vi "Play with rts cts 1002759.vi"(8 "error in (no error)":errorcluster, 11 "Serial open? (y)":bool=TRUE) -> (0 "error out":errorcluster, 1 "RTS control ok?":bool, 3 "PassFail":string, 4 "Comport responsive?":bool, 5 "Comport unresponsive?":bool)   [LabVIEW 2013]
uses:
  NanoArduino/NanoCmds.ctl
  Test Globals/Global 1.vi
panel:
  out "CTS state 0":i16(ring)=-1 items=["Unknown"=-1, "Unasserted"=0, "Asserted"=1]
  out "CTS state 3":i16(ring)=-1 items=["Unknown"=-1, "Unasserted"=0, "Asserted"=1]
  out "Final recv":string
  out "CTS state 2a":i16(ring)=-1 items=["Unknown"=-1, "Unasserted"=0, "Asserted"=1]
  out "CTS state 1a":i16(ring)=-1 items=["Unknown"=-1, "Unasserted"=0, "Asserted"=1]
  out "BYTES RECV WHEN BLOCKING":u32
  in  "Modem port":refnum<visa-resource-name>="COM30"
  out "read buffer no recv":string
  out "VISA resource name out":refnum<visa-resource-name>
  out "read buffer should recv3":string
  out "read buffer no recv 1":string
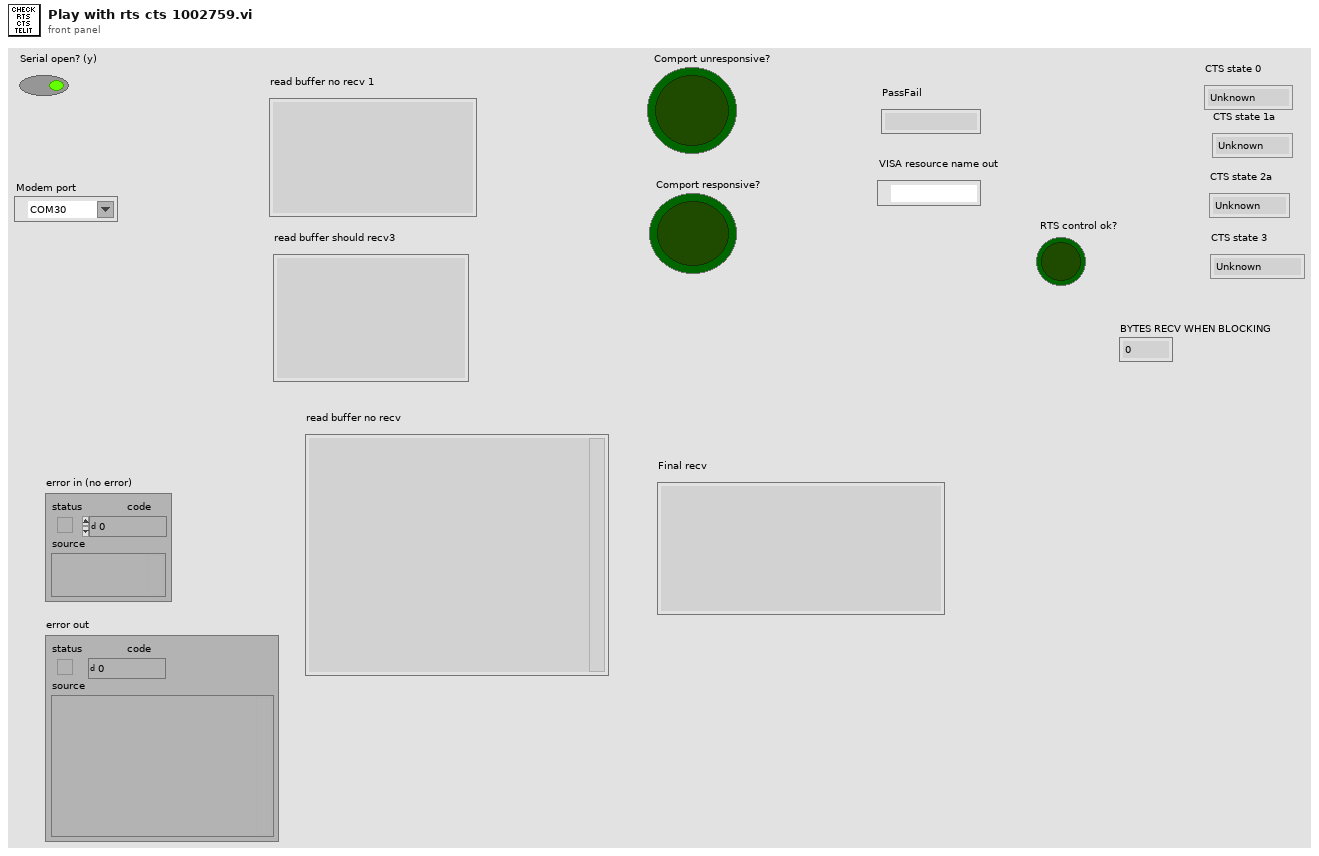
[diagram p1: front panel]
types:
  T1 = typedef "NanoCmds.ctl" = enum16{"Make digital port an output", "Make digital port an input", "Set digital pin high", "Set digital pin low", "Get digital pin state", "Get analog pin voltage", "Get analog pins difference", "Get ohms at analog pin", "Turn on current limit", "Reset Nano device", "Get digital pin state pullup", "Read current", "Initialize", "Power up uut", "Power down uut", "Get uut current draw", "Set ADC volts high", "Set ADC volts low", "Start up uut modem", "Get CTS state", "Get on_nsleep state", "Reset modem", "Get lid state", "Wait for lid closed", "Wait for lid open", "Power up, start, get curr", "Check if X2 shorted", "Power up and start up", "Check X3 shorted", "Get RTS state", "Get DTR state", "Reboot 1002759"}
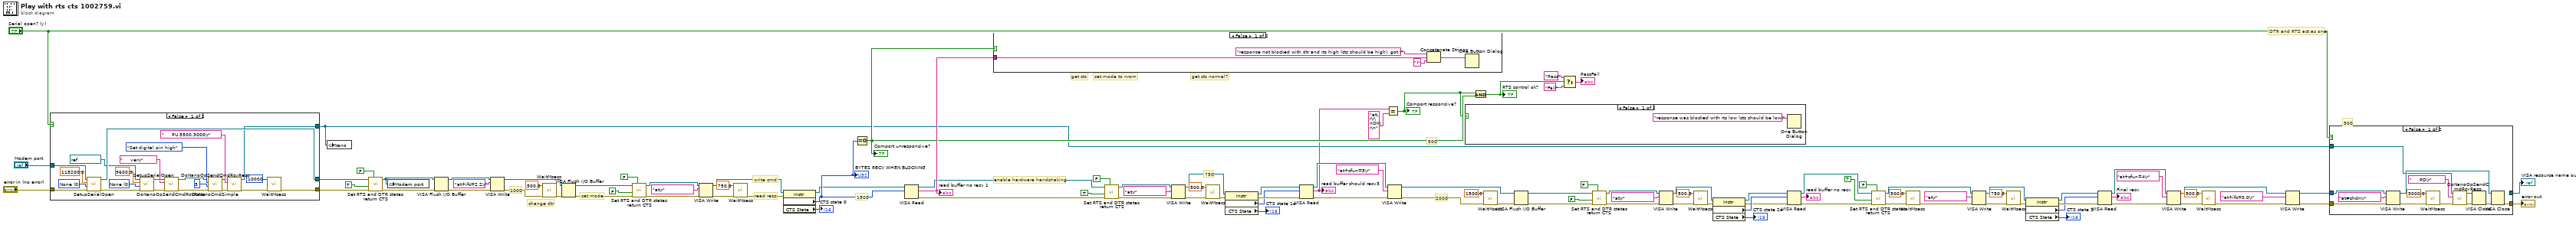
[diagram p0: block diagram]
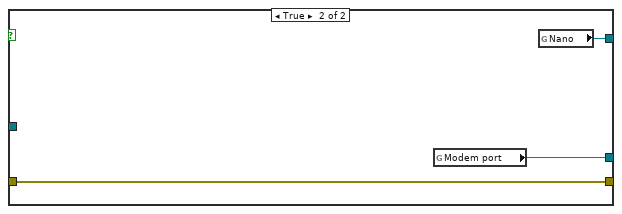
[diagram p3: hidden frame]
diagram:
  # "DTR and RTS act as one"
  # "500"
  # "500"
  # "750"
  # "1000"
  # "2000"
  # "1500"
  # "enable hardware handshaking"
  # "get cts normal?"
  # "set mode to nrom"
  # "read resp"
  # "get cts"
  # "write cmd"
  # "set mode"
  # "change dtr"
  n1 = case shown="False" "Serial open? (y)" {
    tunnel: [w127 w134] -> w15
    tunnel: "Modem port" -> [w131 _]
    tunnel: "error in (no error)" -> [w130 w133]
    tunnel: [w116 w133] -> w16
    tunnel: [w121 w132] -> w4
    frame False {
      w126 = u16 0 items=["None", "XON/XOFF", "RTS/CTS", "XON/XOFF & RTS/CTS", "DTR/DSR", "XON/XOFF & DTR/DSR"] ("flow control (0:none)")
      w128 = u16 0 items=["None", "XON/XOFF", "RTS/CTS", "XON/XOFF & RTS/CTS", "DTR/DSR", "XON/XOFF & DTR/DSR"] ("flow control (0:none)")
      n2 = call "SetupSerialOpen.vi"("error in (no error)"=w130, "flow control (0:none)"=w128, "Baud"=115200.0, "VISA Refnum in"=w131) -> ("error out"=w124:errorcluster, "VISA session"=w127:refnum<visa-resource-name>)  [unwired: 6 in]
      n3 = call "SetupSerialOpen.vi"("error in (no error)"=w124, "flow control (0:none)"=w126, "Baud"=9600.0, "VISA Refnum in"=refnum<visa-resource-name> "COM21") -> ("error out"=w120:errorcluster, "VISA session"=w119:refnum<visa-resource-name>)  [unwired: 6 in]
      n4 = call "DoNanoOpSendCmdRcvResp.vi"("error in (no error)"=w120, "Cmd String"="     ver\r" ("string"), "VISA resource name"=w119) -> ("error out"=w112:errorcluster, "VISA resource name out"=w111:refnum<visa-resource-name>)  [unwired: 2 in, 5 out]
      n5 = call "DoNanoCmdSimple.vi"("error in (no error)"=w112, "Pin 1"=u32 5, "Nano Op"=NanoCmds."Set digital pin high", "VISA resource name"=w111) -> ("error out"=w109:errorcluster, "VISA resource name 2"=w110:refnum<visa-resource-name>)  [unwired: 3 in, 2 out]
      n6 = call "DoNanoOpSendCmdRcvResp.vi"("error in (no error)"=w109, "Cmd String"="     PU,5500,3000\r" ("string"), "VISA resource name"=w110) -> ("error out"=w117:errorcluster, "VISA resource name out"=w121:refnum<visa-resource-name>)  [unwired: 2 in, 5 out]
      n7 = call "WaitMsecs.vi"("error in (no error)"=w117, "Wait Msecs"=u32 10000) -> ("error out"=w116:errorcluster)  [unwired: 9 in]
    }
    frame True {
      n8 = global read "Global 1.vi" "Modem port"() -> (w134:refnum<visa-resource-name>)
      n9 = global read "Global 1.vi" "Nano"() -> (w132:refnum<visa-resource-name>)
    }
  }
  n10 = global write "Global 1.vi" "Nano"(w4) -> ()
  n11 = call "Set RTS and DTR states return CTS.vi"("Assert DTR?"=FALSE, "error in (no error)"=w16, "Assert RTS?"=TRUE, "VISA Refnum in"=w15) -> ("error out"=w13:errorcluster, "Visa ref out"=w14:refnum<visa-resource-name>)  [unwired: 5 in, 1 out]
  n12 = global write "Global 1.vi" "Modem port"(w14) -> ()
  n13 = VISA Flush I/O Buffer(VISA resource name=w14, error in (no error)=w13) -> (VISA resource name out=w94:refnum<visa-resource-name>, error out=w93:errorcluster)  [unwired: 1 in]
  n14 = VISA Write(VISA resource name=w94, write buffer="at+ifc=2,2\r", error in (no error)=w93) -> (VISA resource name out=w2:refnum<visa-resource-name>, error out=w84:errorcluster)  [unwired: 1 out]
  n15 = call "WaitMsecs.vi"("error in (no error)"=w84, "Wait Msecs"=500.0) -> ("error out"=w3:errorcluster)  [unwired: 9 in]
  n16 = VISA Flush I/O Buffer(VISA resource name=w2, error in (no error)=w3) -> (VISA resource name out=w66:refnum<visa-resource-name>, error out=w67:errorcluster)  [unwired: 1 in]
  n17 = call "Set RTS and DTR states return CTS.vi"("Assert DTR?"=FALSE, "error in (no error)"=w67, "Assert RTS?"=FALSE, "VISA Refnum in"=w66) -> ("error out"=w12:errorcluster, "Visa ref out"=w64:refnum<visa-resource-name>)  [unwired: 5 in, 1 out]
  n18 = VISA Write(VISA resource name=w64, write buffer="at\r", error in (no error)=w12) -> (VISA resource name out=w87:refnum<visa-resource-name>, error out=w95:errorcluster)  [unwired: 1 out]
  n19 = call "WaitMsecs.vi"("error in (no error)"=w95, "Wait Msecs"=750.0) -> ("error out"=w8:errorcluster)  [unwired: 9 in]
  n20 = property class="Instr"(reference=w87, error in=w8) -> (reference out=w97:refnum<visa-resource-name>, "Serial Settings:Number of Bytes at Serial Port"=w106:u32, "CTS State"=→"CTS state 0":i16)  [unwired: 1 out]
  "BYTES RECV WHEN BLOCKING" <- w106
  n21 = Equal To 0?(x=w106) -> (x = 0?=w57:bool)
  "Comport unresponsive?" <- w57
  n22 = VISA Read(VISA resource name=w97, byte count=w106) -> (VISA resource name out=w61:refnum<visa-resource-name>, read buffer=w82:string, error out=w62:errorcluster)  [unwired: 1 in, 1 out]
  "read buffer no recv 1" <- w82
  n23 = case shown="False" w57 {
    tunnel: w82 -> [w137 _]
    frame False {
      n24 = Concatenate Strings("response not blocked with dtr and rts high (cts should be high), got (" ("message"), w137, ")" ("string")) -> (w135:string)
      n25 = One Button Dialog(message=w135) -> ()  [unwired: 1 in, 1 out]
    }
    frame True {
    }
  }
  n26 = call "Set RTS and DTR states return CTS.vi"("Assert DTR?"=FALSE, "error in (no error)"=w62, "Assert RTS?"=TRUE, "VISA Refnum in"=w61) -> ("error out"=w11:errorcluster, "Visa ref out"=w56:refnum<visa-resource-name>)  [unwired: 5 in, 1 out]
  n27 = VISA Write(VISA resource name=w56, write buffer="at\r", error in (no error)=w11) -> (VISA resource name out=w39:refnum<visa-resource-name>, error out=w58:errorcluster)  [unwired: 1 out]
  n28 = call "WaitMsecs.vi"("error in (no error)"=w58, "Wait Msecs"=500.0) -> ("error out"=w7:errorcluster)  [unwired: 9 in]
  n29 = property class="Instr"(reference=w39, error in=w7) -> (reference out=w96:refnum<visa-resource-name>, error out=w103:errorcluster, "Serial Settings:Number of Bytes at Serial Port"=w101:u32, "CTS State"=→"CTS state 1a":i16)
  n30 = VISA Read(VISA resource name=w96, byte count=w101, error in (no error)=w103) -> (VISA resource name out=w54:refnum<visa-resource-name>, read buffer=w53:string, error out=w55:errorcluster)  [unwired: 1 out]
  "read buffer should recv3" <- w53
  n31 = Equal?(x=w53, y="at\r\r\nOK\r\n") -> (x = y?=w51:bool)
  "Comport responsive?" <- w51
  n32 = VISA Write(VISA resource name=w54, write buffer="at+cfun=5\r", error in (no error)=w55) -> (VISA resource name out=w49:refnum<visa-resource-name>, error out=w86:errorcluster)  [unwired: 1 out]
  n33 = case shown="False" w51 {
    frame False {
      n34 = One Button Dialog(message="response was blocked with rts low (cts should be low)") -> ()  [unwired: 1 in, 1 out]
    }
    frame True {
    }
  }
  n35 = And(x=w51, y=w57) -> (x .and. y?=w81:bool)
  "RTS control ok?" <- w81
  n36 = call "WaitMsecs.vi"("error in (no error)"=w86, "Wait Msecs"=1500.0) -> ("error out"=w50:errorcluster)  [unwired: 9 in]
  n37 = VISA Flush I/O Buffer(VISA resource name=w49, error in (no error)=w50) -> (VISA resource name out=w42:refnum<visa-resource-name>, error out=w41:errorcluster)  [unwired: 1 in]
  n38 = Select(t="Pass", s=w81, f="Fail") -> (s? t:f=→"PassFail":string)
  n39 = call "Set RTS and DTR states return CTS.vi"("Assert DTR?"=FALSE, "error in (no error)"=w41, "Assert RTS?"=FALSE, "VISA Refnum in"=w42) -> ("error out"=w10:errorcluster, "Visa ref out"=w40:refnum<visa-resource-name>)  [unwired: 5 in, 1 out]
  n40 = VISA Write(VISA resource name=w40, write buffer="at\r", error in (no error)=w10) -> (VISA resource name out=w45:refnum<visa-resource-name>, error out=w48:errorcluster)  [unwired: 1 out]
  n41 = call "WaitMsecs.vi"("error in (no error)"=w48, "Wait Msecs"=500.0) -> ("error out"=w6:errorcluster)  [unwired: 9 in]
  n42 = property class="Instr"(reference=w45, error in=w6) -> (reference out=w90:refnum<visa-resource-name>, error out=w89:errorcluster, "Serial Settings:Number of Bytes at Serial Port"=w91:u32, "CTS State"=→"CTS state 2a":i16)
  n43 = VISA Read(VISA resource name=w90, byte count=w91, error in (no error)=w89) -> (VISA resource name out=w33:refnum<visa-resource-name>, read buffer=→"read buffer no recv":string, error out=w34:errorcluster)  [unwired: 1 out]
  n44 = call "Set RTS and DTR states return CTS.vi"("Assert DTR?"=FALSE, "error in (no error)"=w34, "Assert RTS?"=TRUE, "VISA Refnum in"=w33) -> ("error out"=w31:errorcluster, "Visa ref out"=w20:refnum<visa-resource-name>)  [unwired: 5 in, 1 out]
  n45 = call "WaitMsecs.vi"("error in (no error)"=w31, "Wait Msecs"=500.0) -> ("error out"=w21:errorcluster)  [unwired: 9 in]
  n46 = VISA Write(VISA resource name=w20, write buffer="at\r", error in (no error)=w21) -> (VISA resource name out=w19:refnum<visa-resource-name>, error out=w22:errorcluster)  [unwired: 1 out]
  n47 = call "WaitMsecs.vi"("error in (no error)"=w22, "Wait Msecs"=750.0) -> ("error out"=w5:errorcluster)  [unwired: 9 in]
  n48 = property class="Instr"(reference=w19, error in=w5) -> (reference out=w29:refnum<visa-resource-name>, error out=w30:errorcluster, "Serial Settings:Number of Bytes at Serial Port"=w28:u32, "CTS State"=→"CTS state 3":i16)
  n49 = VISA Read(VISA resource name=w29, byte count=w28, error in (no error)=w30) -> (VISA resource name out=w25:refnum<visa-resource-name>, read buffer=→"Final recv":string, error out=w26:errorcluster)  [unwired: 1 out]
  n50 = VISA Write(VISA resource name=w25, write buffer="at+cfun=4\r", error in (no error)=w26) -> (VISA resource name out=w74:refnum<visa-resource-name>, error out=w70:errorcluster)  [unwired: 1 out]
  n51 = call "WaitMsecs.vi"("error in (no error)"=w70, "Wait Msecs"=500.0) -> ("error out"=w69:errorcluster)  [unwired: 9 in]
  n52 = VISA Write(VISA resource name=w74, write buffer="at+ifc=0,0\r", error in (no error)=w69) -> (VISA resource name out=w73:refnum<visa-resource-name>, error out=w75:errorcluster)  [unwired: 1 out]
  n53 = case shown="False" "Serial open? (y)" {
    tunnel: w75 -> [w143 w154]
    tunnel: w73 -> [w144 w153]
    tunnel: [w151 w154] -> w76
    tunnel: [_ w153] -> w77
    tunnel: w4 -> [w140 _]
    frame False {
      n54 = VISA Write(VISA resource name=w144, write buffer="at#shdn\r", error in (no error)=w143) -> (VISA resource name out=w141:refnum<visa-resource-name>, error out=w147:errorcluster)  [unwired: 1 out]
      n55 = call "WaitMsecs.vi"("error in (no error)"=w147, "Wait Msecs"=3000.0) -> ("error out"=w142:errorcluster)  [unwired: 9 in]
      n56 = call "DoNanoOpSendCmdRcvResp.vi"("error in (no error)"=w142, "Cmd String"="     PD\r" ("string"), "VISA resource name"=w140) -> ("error out"=w149:errorcluster, "VISA resource name out"=w148:refnum<visa-resource-name>)  [unwired: 2 in, 5 out]
      n57 = VISA Close(VISA resource name=w148, error in (no error)=w149) -> (error out=w152:errorcluster)
      n58 = VISA Close(VISA resource name=w141, error in (no error)=w152) -> (error out=w151:errorcluster)
    }
    frame True {
    }
  }
  "error out" <- w76
  "VISA resource name out" <- w77
